vi "JOYSTICK Teleop.vi"(10 "Match Info":T2={"Autonomous Elapsed Seconds"=0.0, "TeleOp Elapsed Seconds"=0.0, "Disabled Elapsed Seconds"=0.0, "Visited Autonomous"=FALSE, "Visited TeleOp"=FALSE, "Visited Disabled"=FALSE, "Autonomous Settings"={"Autonomous Style"=enum."Independent", "VI Refnum"=refnum}}, 11 "Call Context":T3) -> ()   [LabVIEW 2020]
doc: "This VI is called for each TeleOp packet received from the DS where the robot is not disabled. It is often used to read from the joysticks and update I/O or to update setpoints for timed control loops. It should complete and return within 20 milliseconds or it may miss DS packets."
uses:
  <vilib>/Rock Robotics/Network Tables/NT Write Boolean.vi
  Systems/Game Controller/Global_SEN_Data Out.vi
  Systems/Game Controller/GameController_SEN.lvlib
  Systems/SwerveDrive/Global_CMD_ACT_Data In.vi
  Systems/SwerveDrive/SwerveDrive_ACT.lvlib
  Shared Code/TypeDefs/ENUM_Swerve_CMD_Mode Select.ctl
  Shared Code/TypeDefs/Cluster_CMD_Direction Data.ctl
  Systems/SwerveDrive/Cluster_CMD_ACT_Data.ctl
  Shared Code/TypeDefs/Dial_Compase heading unit circle CCW positive.ctl
  Shared Code/TypeDefs/Level_Velocity plus-minus 1.ctl
  Shared Code/TypeDefs/Cluster_Module Velocity-Direction-Rotations.ctl
  Shared Code/TypeDefs/Cluster_X-Y.ctl
  Systems/PigeonIMU/Global_CMD_SEN_Data In.vi
  Systems/PigeonIMU/PigeonIMU_SEN.lvlib
  Systems/PigeonIMU/Cluster_CMD_SEN_Data.ctl
  Systems/Joystick Controller/Global_SEN_Data Out.vi
  Systems/Joystick Controller/JoystickController_SEN.lvlib
  Type Defs/NUM_Rotate Input.ctl
  <vilib>/Rock Robotics/WPI/DriverStation/WPI_DriverStationMatch Info.ctl
  <vilib>/Rock Robotics/WPI/DriverStation/WPI_DriverStationDerivedRobotMode.ctl
panel:
  in  "Translation Speed (ft/s)":dbl=10.0 format="%#_13g"
  out "Drive Mode":T1
  out "POV":i16
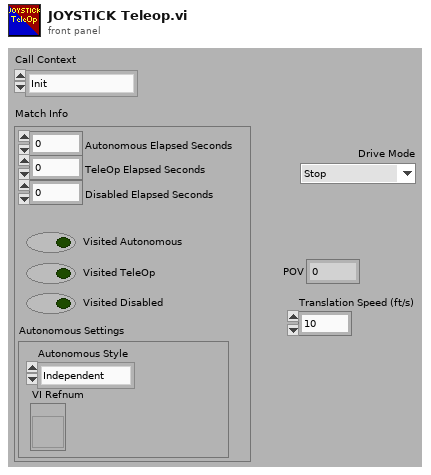
[diagram p1: front panel]
types:
  T1 = typedef "ENUM_Swerve_CMD_Mode Select.ctl" = enum16{"Stop", "Move", "Turret Manual"}
  T2 = typedef "WPI_DriverStationMatch Info.ctl" = cluster{"Autonomous Elapsed Seconds":dbl, "TeleOp Elapsed Seconds":dbl, "Disabled Elapsed Seconds":dbl, "Visited Autonomous":bool, "Visited TeleOp":bool, "Visited Disabled":bool, "Autonomous Settings":cluster{"Autonomous Style":enum16{"Iterative", "Independent"}, "VI Refnum":refnum<vi>}}
  T3 = typedef "WPI_DriverStationDerivedRobotMode.ctl" = enum16{"Init", "Execute", "Stop"}
  T4 = typedef "PigeonIMU_SEN.lvlib/Cluster_CMD_SEN_Data.ctl" = cluster{"Reset":bool, "Disable":bool}
  T5 = typedef "Cluster_Module Velocity-Direction-Rotations.ctl" = cluster{"Velocity":T6, "Angle":T7, "Rotations Count":dbl}
  T6 = typedef "Level_Velocity plus-minus 1.ctl" = dbl
  T7 = typedef "Dial_Compase heading unit circle CCW positive.ctl" = dbl
  T8 = typedef "SwerveDrive_ACT.lvlib/Cluster_CMD_ACT_Data.ctl" = cluster{"Mode":T1, "Direction":T9, "Orientation Robot(t) Field(f)":bool, "Max Translation Speed (ft/sec)":dbl, "Rotation Reduction 1-0":dbl, "Rotation Center From Robot Center":T11}
  T9 = typedef "Cluster_CMD_Direction Data.ctl" = cluster{"Traverse":T5, "Rotate(Yaw) CCW 1 CW -1":T10}
  T10 = typedef "NUM_Rotate Input.ctl" = dbl
  T11 = typedef "Cluster_X-Y.ctl" = cluster{"X":dbl, "Y":dbl}
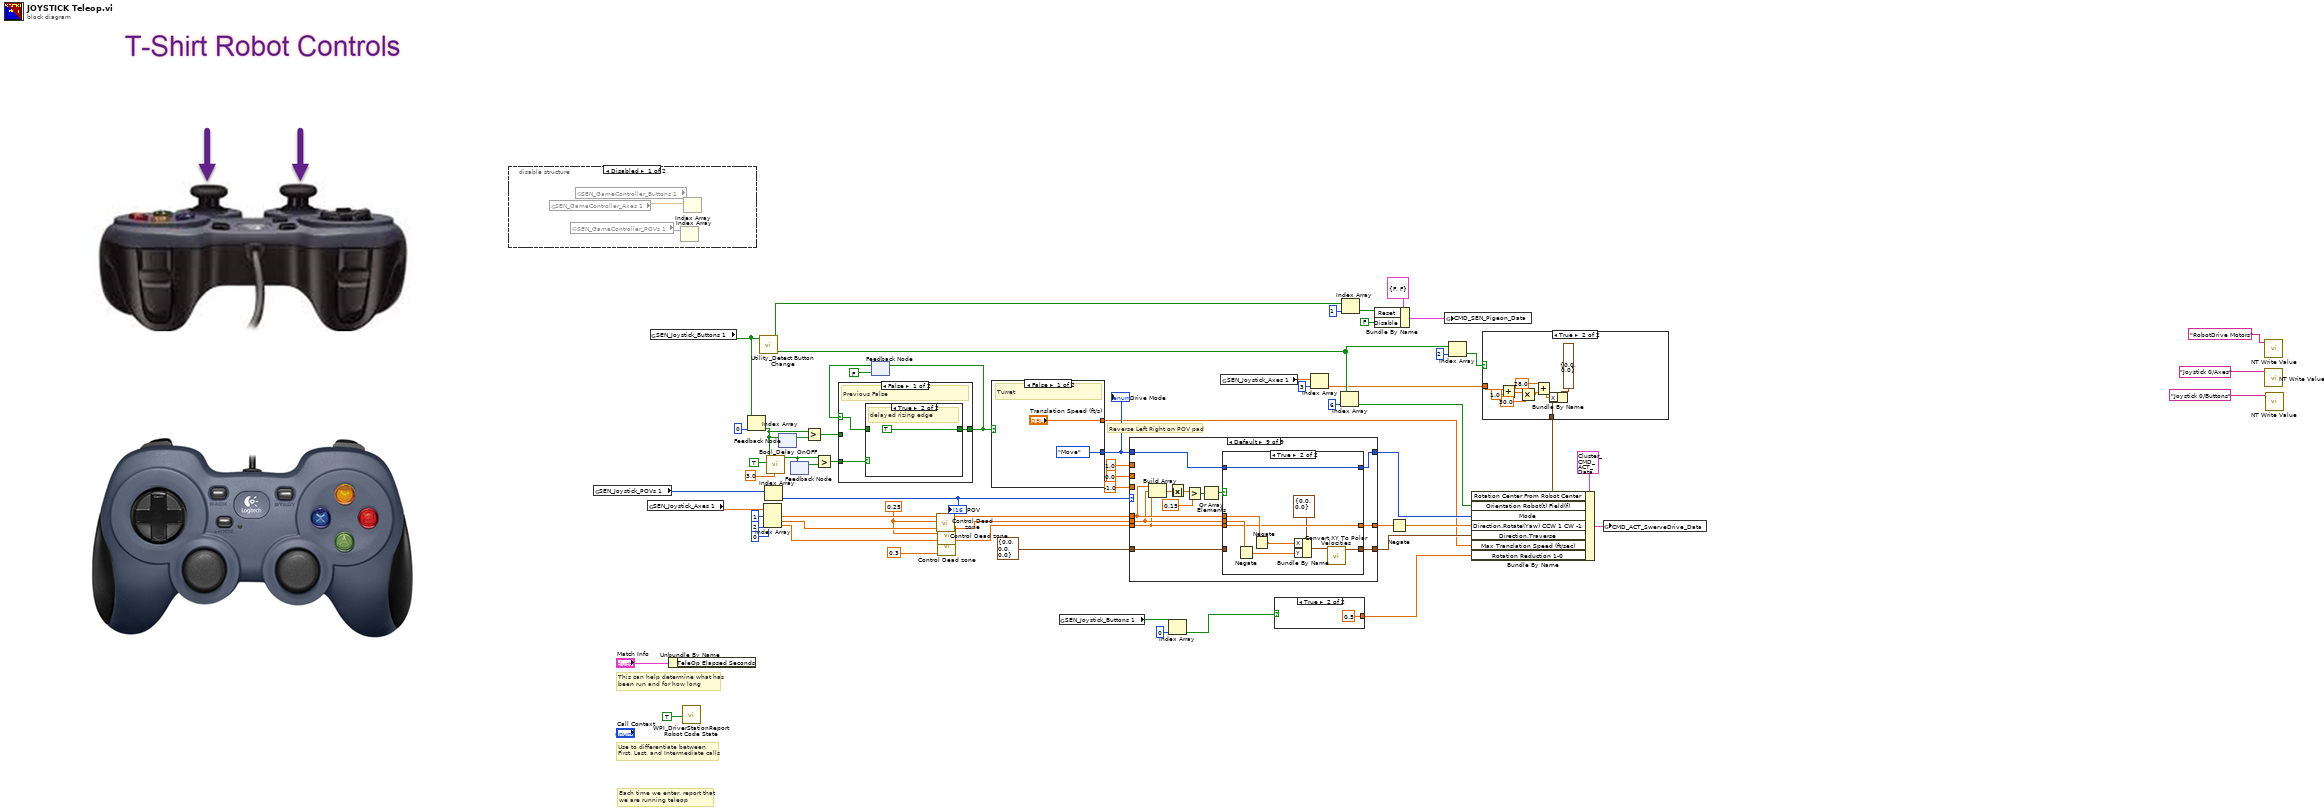
[diagram p0: block diagram]
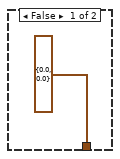
[diagram p2: hidden frame]
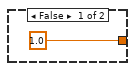
[diagram p3: hidden frame]
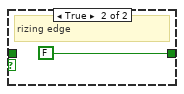
[diagram p6: hidden frame]
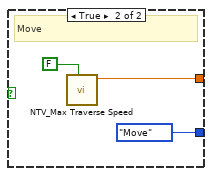
[diagram p7: hidden frame]
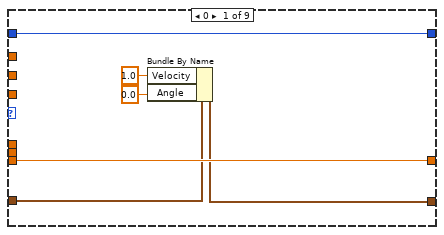
[diagram p9: hidden frame]
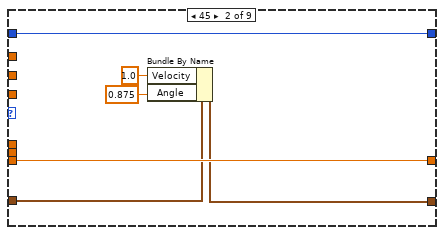
[diagram p10: hidden frame]
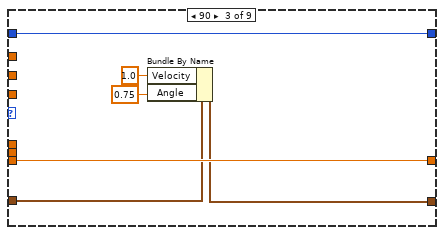
[diagram p11: hidden frame]
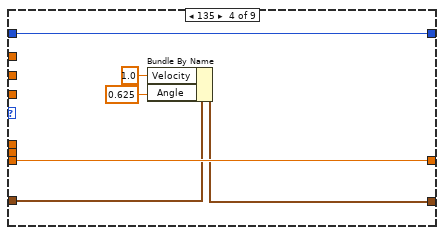
[diagram p12: hidden frame]
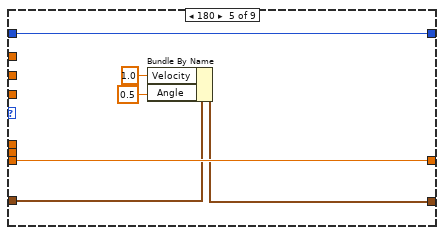
[diagram p13: hidden frame]
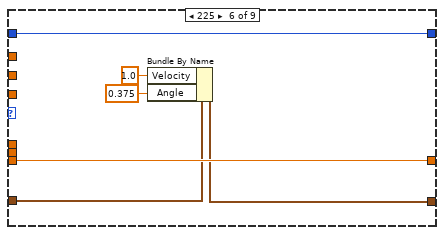
[diagram p14: hidden frame]
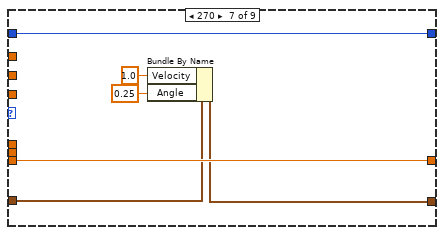
[diagram p15: hidden frame]
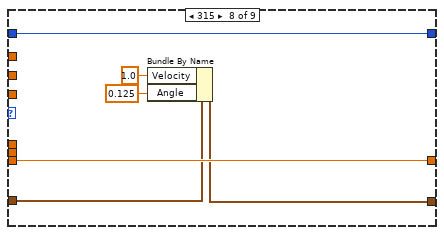
[diagram p16: hidden frame]
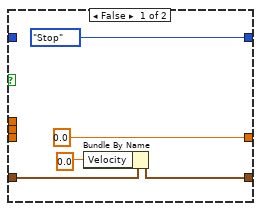
[diagram p17: hidden frame]
diagram:
  w40 = 0.25 ("y")
  # "Reverse Left Right on POV pad"
  # "Each time we enter, report that\nwe are running teleop"
  # "Use to differentiate between\nFirst, Last, and Intermediate calls"
  # "This can help determine what has\nbeen run and for how long"
  n1 = disable-structure shown="Disabled" {
    frame Disabled {
      n2 = global read "Global_SEN_Data Out.vi" "SEN_GameController_Axes 1"() -> (w65:dbl[])
      n3 = global read "Global_SEN_Data Out.vi" "SEN_GameController_POVs 1"() -> (w64:i16[])
      n4 = global read "Global_SEN_Data Out.vi" "SEN_GameController_Buttons 1"() -> ()  [unwired: 1 out]
      n5 = Index Array(array=w64) -> ()  [unwired: 1 in, 1 out]
      n6 = Index Array(array=w65) -> ()  [unwired: 1 in, 1 out]
    }
    frame Enabled {
    }
  }
  n7 = global read "Global_SEN_Data Out.vi" "SEN_Joystick_POVs 1"() -> (w14:i16[])
  n8 = global read "Global_SEN_Data Out.vi" "SEN_Joystick_Axes 1"() -> (w10:dbl[])
  n9 = global read "Global_SEN_Data Out.vi" "SEN_Joystick_Buttons 1"() -> (w15:bool[])
  n10 = Unbundle By Name("Match Info") -> ()  [unwired: 1 out]
  n11 = call <vilib>:"WPI_DriverStationReport Robot Code State.vi"("TeleOp"=TRUE ("Autonomous")) -> ()  [unwired: 10 in, 1 out]
  n12 = Index Array(array=w15, index=0) -> (element=w25:bool)
  n13 = call "Utility_Detect Button Change.vi"("HW_Joystick_Buttons"=w15) -> ("Toggle On Rising Out"=w18:bool[], "Value Out"=w32:bool[])  [unwired: 6 in, 3 out]
  n14 = Index Array(array=w10, index #1=1 ("index"), index #2=2 ("index"), index #3=0 ("index")) -> (element #1=w49:dbl, element #2=w42:dbl, element #3=w41:dbl)
  n15 = Index Array(array=w14) -> (element=w58:i16)  [unwired: 1 in]
  "POV" <- w58
  n16 = call "Bool_Delay OnOFF.vi"("Delay Time(S)"=3.0, "Delay On(t) Off(f)"=TRUE, "Input"=w25) -> ("Output"=w26:bool)  [unwired: 7 in, 1 out]
  n17 = feedback #1() -> (w24:bool)  [unwired: 1 in]
  n18 = feedback-in #1(w25) -> ()
  n19 = feedback-in #2(w26) -> ()
  n20 = feedback #2() -> (w22:bool)  [unwired: 1 in]
  n21 = Greater?(x=w25, y=w24) -> (0:w23:bool)
  n22 = Greater?(x=w26, y=w22) -> (0:w21:bool)
  n23 = feedback #3(FALSE) -> (w30:bool)
  n24 = case shown="False" w30 {
    selector: w30 -> [w67 w72]
    tunnel: [w68 w73] -> w29
    tunnel: w23 -> [_ w71]
    tunnel: w21 -> [w66 _]
    frame False {
      # "Previous False"
      n25 = case shown="True" w66 {
        tunnel: [w69 TRUE] -> w68
        tunnel: w67 -> [w69 _]
        frame False {
        }
        frame True {
          # "delayed rizing edge"
        }
      }
    }
    frame True {
      # "Previous True"
      n26 = case shown="False" w71 {
        tunnel: [w74 FALSE] -> w73
        tunnel: w72 -> [w74 _]
        frame False {
          # "not Rizing"
        }
        frame True {
          # "rizing edge"
        }
      }
    }
  }
  n27 = feedback-in #3(w29) -> ()
  n28 = call "Control Dead zone.vi"("dead zone"=w40, "control Value"=w49) -> ("output Value"=w48:dbl)  [unwired: 9 in]
  n29 = call "Control Dead zone.vi"("dead zone"=w40, "control Value"=w42) -> ("output Value"=w44:dbl)  [unwired: 9 in]
  n30 = call "Control Dead zone.vi"("dead zone"=0.3 ("y"), "control Value"=w41) -> ("output Value"=w43:dbl)  [unwired: 9 in]
  n31 = case shown="False" w29 {
    tunnel: [ENUM_Swerve_CMD_Mode_Select."Move" ("Mode") ENUM_Swerve_CMD_Mode_Select."Move" ("Mode")] -> w54
    tunnel: ["Translation Speed (ft/s)" w78] -> w33
    frame False {
      # "Turret"
    }
    frame True {
      # "Move"
      n32 = call "NTV_Max Traverse Speed.vi"("Read(f) Write(t)"=FALSE) -> ("MAx Traverse Speed FPS Out"=w78:dbl)  [unwired: 10 in]
    }
  }
  "Drive Mode" <- w54
  n33 = global read "Global_SEN_Data Out.vi" "SEN_Joystick_Buttons 1"() -> (w11:bool[])
  n34 = case shown="Default" w58 {
    tunnel: 1.0 ("Direction.Travers Left 1 Right -1") -> [_ _ _ _ _ _ _ _ _]
    tunnel: 0.0 ("Direction.Travers Left 1 Right -1") -> [_ _ _ _ _ _ _ _ _]
    tunnel: -1.0 ("Direction.Travers Left 1 Right -1") -> [_ _ _ _ _ _ _ _ _]
    tunnel: w54 -> [w86 w92 w98 w104 w110 w116 w122 w128 w141]
    tunnel: [w86 w92 w98 w104 w110 w116 w122 w128 w140] -> w53
    tunnel: w48 -> [_ _ _ _ _ _ _ _ w138]
    tunnel: w44 -> [_ _ _ _ _ _ _ _ w137]
    tunnel: w43 -> [w85 w91 w97 w103 w109 w115 w121 w127 w136]
    tunnel: [w85 w91 w97 w103 w109 w115 w121 w127 w139] -> w50
    tunnel: T5 {"Velocity"=0.0, "Angle"=0.0, "Rotations Count"=0.0} ("Polar Out") -> [w84 w90 w96 w102 w108 w114 w120 w126 w130]
    tunnel: [w81 w87 w93 w99 w105 w111 w117 w123 w129] -> w45
    frame 0 {
      n35 = Bundle By Name(cluster=w84, "Velocity"=T6 1.0, "Angle"=T7 0.0) -> (w81:T5)
    }
    frame 45 {
      n36 = Bundle By Name(cluster=w90, "Velocity"=T6 1.0, "Angle"=T7 0.875) -> (w87:T5)
    }
    frame 90 {
      n37 = Bundle By Name(cluster=w96, "Velocity"=T6 1.0, "Angle"=T7 0.75) -> (w93:T5)
    }
    frame 135 {
      n38 = Bundle By Name(cluster=w102, "Velocity"=T6 1.0, "Angle"=T7 0.625) -> (w99:T5)
    }
    frame 180 {
      n39 = Bundle By Name(cluster=w108, "Velocity"=T6 1.0, "Angle"=T7 0.5) -> (w105:T5)
    }
    frame 225 {
      n40 = Bundle By Name(cluster=w114, "Velocity"=T6 1.0, "Angle"=T7 0.375) -> (w111:T5)
    }
    frame 270 {
      n41 = Bundle By Name(cluster=w120, "Velocity"=T6 1.0, "Angle"=T7 0.25) -> (w117:T5)
    }
    frame 315 {
      n42 = Bundle By Name(cluster=w126, "Velocity"=T6 1.0, "Angle"=T7 0.125) -> (w123:T5)
    }
    frame Default {
      n43 = Build Array(w138, w137, w136) -> (w135:dbl[])
      n44 = Absolute Value(x=w135) -> (abs(x)=w131:dbl[])
      n45 = Greater?(x=w131, y=0.15 ("upper limit")) -> (0:w133:bool[])
      n46 = Or Array Elements(Boolean array=w133) -> (logical OR=w132:bool)
      n47 = case shown="True" w132 {
        tunnel: w141 -> [_ w153]
        tunnel: [ENUM_Swerve_CMD_Mode_Select."Stop" ("Mode") w153] -> w140
        tunnel: w138 -> [_ w155]
        tunnel: w137 -> [_ w154]
        tunnel: w136 -> [_ w152]
        tunnel: [0.0 ("f") w152] -> w139
        tunnel: w130 -> [w144 _]
        tunnel: [w145 w149] -> w129
        frame False {
          n48 = Bundle By Name(cluster=w144, "Velocity"=T6 0.0) -> (w145:T5)
        }
        frame True {
          n49 = Negate(x=w154) -> (-x=w148:dbl)
          n50 = Negate(x=w155) -> (-x=w147:dbl)
          n51 = Bundle By Name(cluster=T11 {"X"=0.0, "Y"=0.0} ("XY Velocities"), "X"=w147, "Y"=w148) -> (w151:T11)
          n52 = call "Convert XY To Polar Velocities.vi"("XY Velocities"=w151) -> ("Polar Out"=w149:T5)  [unwired: 10 in]
        }
      }
    }
  }
  n53 = Index Array(array=w11, index=0) -> (element=w19:bool)
  n54 = global read "Global_SEN_Data Out.vi" "SEN_Joystick_Axes 1"() -> (w8:dbl[])
  n55 = case shown="True" w19 {
    tunnel: [1.0 0.5] -> w20
    frame False {
    }
    frame True {
    }
  }
  n56 = Index Array(array=w8, index=3) -> (element=w6:dbl)
  n57 = Index Array(array=w18, index=6) -> (element=w38:bool)
  n58 = Index Array(array=w32, index=1) -> (element=w35:bool)
  n59 = Bundle By Name(cluster=T4 {"Reset"=FALSE, "Disable"=FALSE} ("CMD_SEN_Pigeon_Data"), "Reset"=w35, "Disable"=FALSE) -> (w36:T4)
  n60 = Negate(x=w50) -> (-x=w47:dbl)
  n61 = global write "Global_CMD_SEN_Data In.vi" "CMD_SEN_Pigeon_Data"(w36) -> ()
  n62 = Index Array(array=w18, index=2) -> (element=w17:bool)
  n63 = case shown="True" w17 {
    tunnel: [T11 {"X"=0.0, "Y"=0.0} ("Rotation Center From Robot Center") w159] -> w16
    tunnel: w6 -> [_ w167]
    frame False {
    }
    frame True {
      n64 = Add(x=w167, y=1.0) -> (x+y=w165:dbl)
      n65 = Multiply(x=w165, y=30.0) -> (x*y=w163:dbl)
      n66 = Add(x=28.0, y=w163) -> (x+y=w161:dbl)
      n67 = Bundle By Name(cluster=T11 {"X"=0.0, "Y"=0.0} ("Rotation Center From Robot Center"), "X"=w161) -> (w159:T11)
    }
  }
  n68 = Bundle By Name(cluster=T8 {"Mode"=enum."Stop", "Direction"={"Traverse"={"Velocity"=0.0, "Angle"=0.0, "Rotations Count"=0.0}, "Rotate(Yaw) CCW 1 CW -1"=0.0}, "Orientation Robot(t) Field(f)"=FALSE, "Max Translation Speed (ft/sec)"=0.0, "Rotation Reduction 1-0"=0.0, "Rotation Center From Robot Center"={"X"=0.0, "Y"=0.0}} ("CMD_ACT_Template_Data"), "Rotation Center From Robot Center"=w16, "Orientation Robot(t) Field(f)"=w38, "Mode"=w53, "Direction.Rotate(Yaw) CCW 1 CW -1"=w47, "Direction.Traverse"=w45, "Max Translation Speed (ft/sec)"=w33, "Rotation Reduction 1-0"=w20) -> (w51:T8)
  n69 = global write "Global_CMD_ACT_Data In.vi" "CMD_ACT_SwerveDrive_Data"(w51) -> ()
  n70 = call-poly <vilib>:"NT Write Value.vi"("name"="RobotDrive Motors" ("Name")) -> ()  [unwired: 10 in, 1 out]
  n71 = call-poly <vilib>:"NT Write Value.vi"("name"="Joystick 0/Axes" ("Name")) -> ()  [unwired: 10 in, 1 out]
  n72 = call-poly <vilib>:"NT Write Value.vi"("name"="Joystick 0/Buttons" ("Name")) -> ()  [unwired: 10 in, 1 out]
